vi "drivetrain_shift_state_store.vi"(10 "data_store_mode":enum16{"Set", "Get"}(ring), 11 "gear shift state":T1) -> (3 "gear shift state out":T1)   [LabVIEW 2011]
uses:
  gear_shift_state.ctl
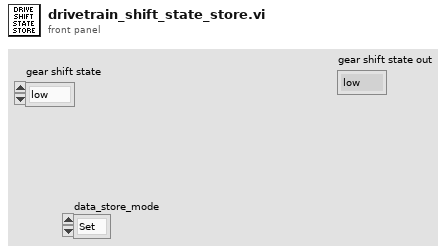
[diagram p1: front panel]
types:
  T1 = typedef "gear_shift_state.ctl" = enum16{"low", "high"}
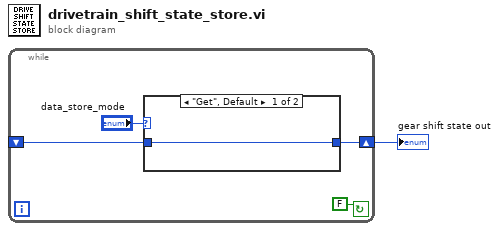
[diagram p0: block diagram]
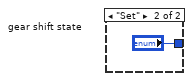
[diagram p2: hidden frame]
diagram:
  n1 = while {
    shift-right: [w3] -> w1
    shift-left: _ -> [w2]
    stop <- FALSE continue-if-true
    n2 = case shown="\"Get\", Default" "data_store_mode" {
      tunnel: [w6 "gear shift state"] -> w3
      tunnel: w2 -> [w6 _]
      frame "Get", Default {
      }
      frame "Set" {
      }
    }
  }
  "gear shift state out" <- w1
